vi "Compare FPGA.vi"(8 "error in (no error)":errorcluster, 10 "UDV Container":refnum<k21>[](array[refnum]), 11 "FPGA in":T1[](array[typedef]) {"UDVs"."To FPGA"."VS ref" format="%.0x"; "UDVs"."From FPGA"."VS ref" format="%.0x"; "VS ref" format="%.0x"; "Output Data"."BD Refs"."Data Reference" format="%.0x"; "Input Data"."BD Refs"."Data Reference" format="%.0x"}) -> (0 "error out":errorcluster, 3 "FPGA out":T1[](array[typedef]) {"UDVs"."To FPGA"."VS ref" format="%.0x"; "UDVs"."From FPGA"."VS ref" format="%.0x"; "VS ref" format="%.0x"; "Output Data"."BD Refs"."Data Reference" format="%.0x"; "Input Data"."BD Refs"."Data Reference" format="%.0x"})   [LabVIEW 2019, in "SEECD Engine.lvlib"]
uses:
  SEECD Engine.lvlib
  Type Defs/FPGA Data.ctl
  <vilib>/NI VeriStand/Custom Device API/Custom Device Item Ref.ctl
  Type Defs/Input Data.ctl
  <vilib>/NI VeriStand/Custom Device API/Block Data Reference.ctl
  <vilib>/NI VeriStand/Custom Device API/Data Reference.ctl
  Type Defs/Output Data.ctl
  Type Defs/UDV Data.ctl
  Type Defs/UDV Data Type.ctl
  Type Defs/FXP Config.ctl
  Shared/Globals/Error Strings.vi
  <resource>/objmgr/ni.var.rc
  <vilib>/NI VeriStand/Custom Device API/Custom Device API.lvlib
  Shared/SEECD Shared.lvlib
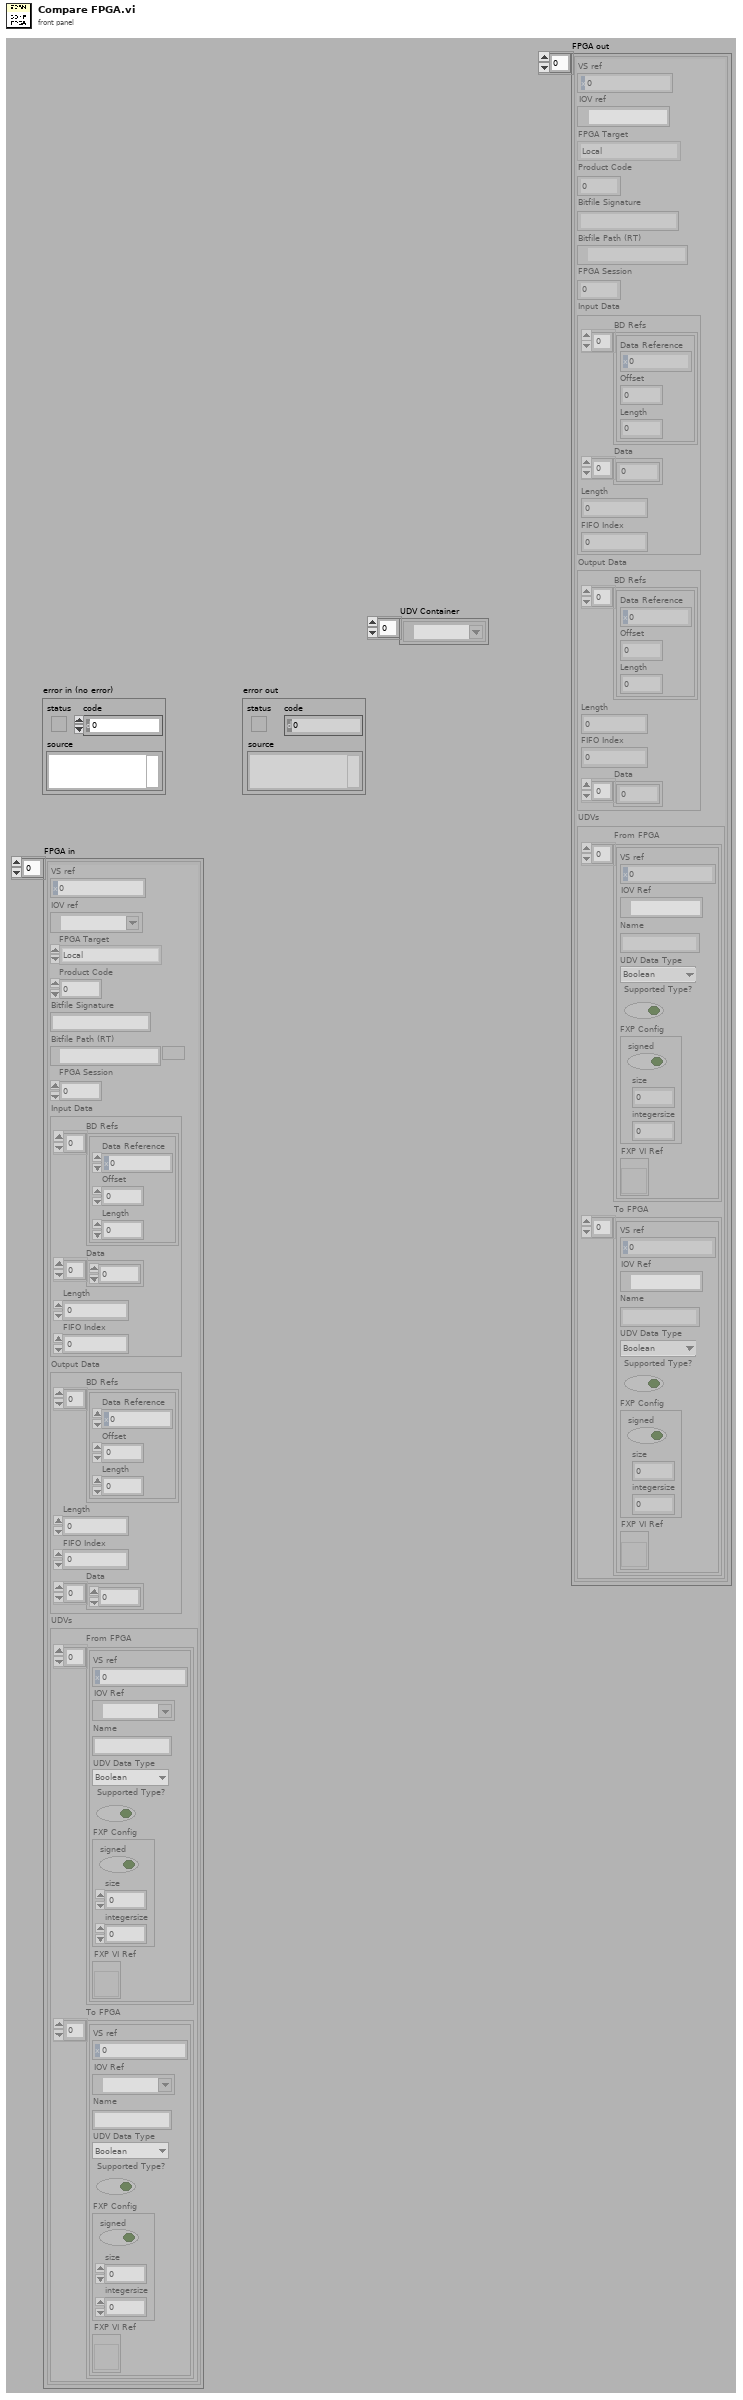
[diagram p1: front panel]
types:
  T1 = typedef "SEECD Engine.lvlib/FPGA Data.ctl" = cluster{"VS ref":T2, "IOV ref":refnum<k21>, "FPGA Target":enum16{"Local", "EtherCAT"}, "Product Code":u32, "Bitfile Signature":string, "Bitfile Path (RT)":path, "FPGA Session":u32, "Input Data":T3, "Output Data":T6, "UDVs":cluster{"From FPGA":T7[], "To FPGA":T7[]}}
  T2 = typedef "Custom Device API.lvlib/Custom Device Item Ref.ctl" = u64
  T3 = typedef "SEECD Engine.lvlib/Input Data.ctl" = cluster{"BD Refs":T4[], "Data":dbl[], "Length":i32, "FIFO Index":i32}
  T4 = typedef "Custom Device API.lvlib/Block Data Reference.ctl" = cluster{"Data Reference":T5, "Offset":u64, "Length":u64}
  T5 = typedef "Custom Device API.lvlib/Data Reference.ctl" = i32
  T6 = typedef "SEECD Engine.lvlib/Output Data.ctl" = cluster{"BD Refs":T4[], "Length":i32, "FIFO Index":i32, "Data":dbl[]}
  T7 = typedef "SEECD Engine.lvlib/UDV Data.ctl" = cluster{"VS ref":T2, "IOV Ref":refnum<k21>, "Name":string, "UDV Data Type":T8, "Supported Type?":bool, "FXP Config":T9, "FXP VI Ref":refnum<vi>}
  T8 = typedef "SEECD Engine.lvlib/UDV Data Type.ctl" = enum16{"Boolean", "Fixed Point", "Int8", "Int16", "Int32", "Int64", "U32 Bit Field", "UInt8", "UInt16", "UInt32", "UInt64", "Other", "DBL", "SGL"}
  T9 = typedef "SEECD Engine.lvlib/FXP Config.ctl" = cluster{"signed":bool, "size":u32, "integersize":i32}
  T10 = typedef "Custom Device API.lvlib/Custom Device Item Info.ctl" = cluster{"Name":string, "Is Channel":bool, "GUID":string, "Is Waveform":bool}
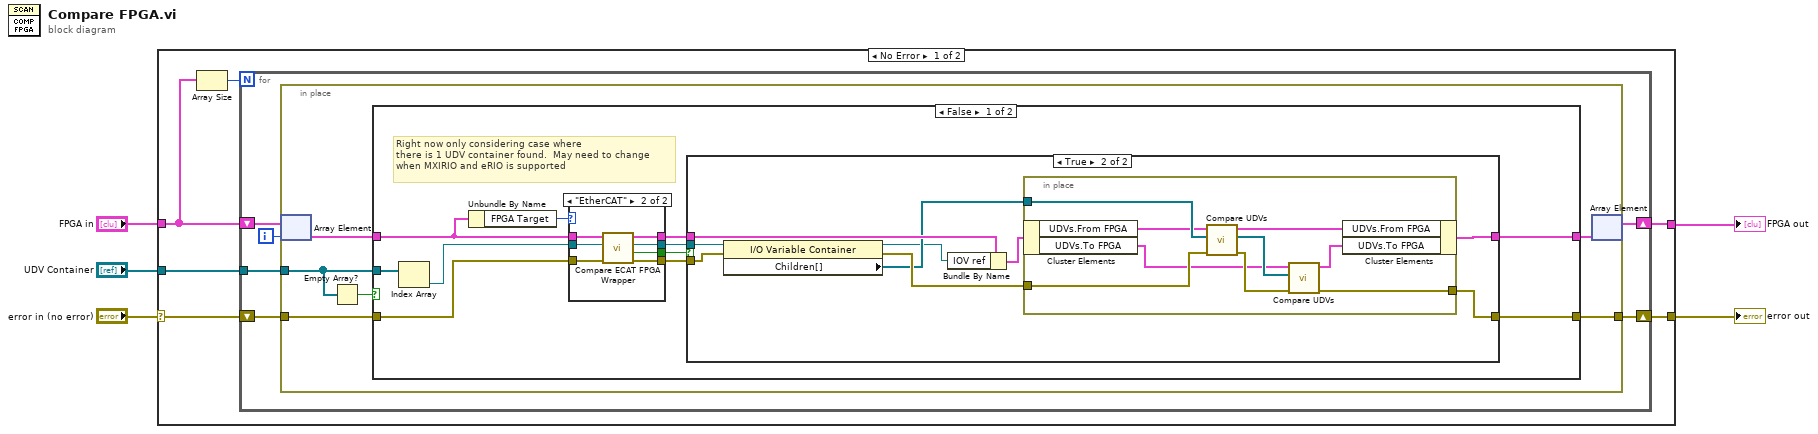
[diagram p0: block diagram]
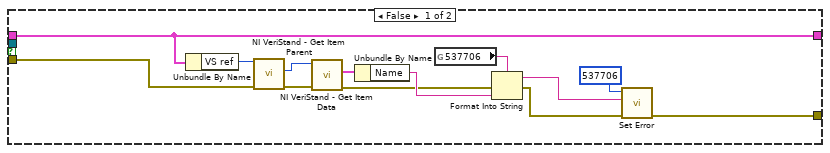
[diagram p2: hidden frame]
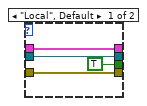
[diagram p3: hidden frame]
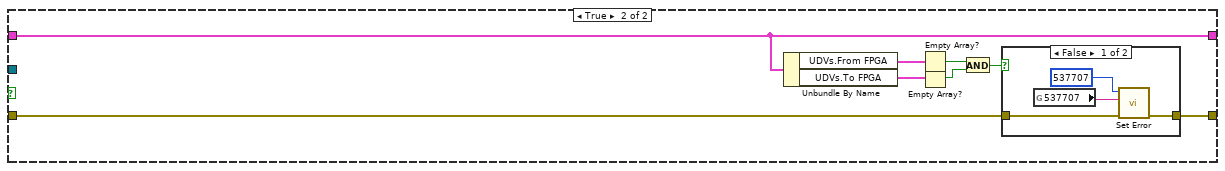
[diagram p4: hidden frame]
diagram:
  n1 = case shown="No Error" "error in (no error)" {
    selector: "error in (no error)" -> [w11 w91]
    tunnel: [w9 w91] -> w4
    tunnel: "FPGA in" -> [w7 w90]
    tunnel: "UDV Container" -> [w10 _]
    tunnel: [w6 w90] -> w1
    frame No Error {
      n2 = Array Size(array=w7) -> (size(s)=w8:i32)
      n3 = for {
        N: w8 -> [_]
        tunnel: w10 -> [w17]
        shift-right: [w13] -> w9
        shift-left: w11 -> [w16]
        shift-right: [w12] -> w6
        shift-left: w7 -> [w15]
        i -> [w14]
        n4 = in-place {
          in-place-border: w17 -> [w22]
          in-place-border: w16 -> [w21]
          in-place-border: [w18] -> w13
          n5 = in-place-array #1(w15, w14) -> (w20:T1)
          n6 = Empty Array?(array=w22) -> (empty?=w23:bool)
          n7 = case shown="False" w23 {
            tunnel: w20 -> [w32 w82]
            tunnel: w22 -> [w31 _]
            tunnel: w21 -> [w29 w83]
            tunnel: [w25 w82] -> w19
            tunnel: [w24 w84] -> w18
            frame False {
              # "Right now only considering case where\nthere is 1 UDV container found.  May need to change\nwhen MXIRIO and eRIO is supported"
              n8 = Index Array(array=w31) -> (element=w30:refnum<k21>)  [unwired: 1 in]
              n9 = Unbundle By Name(w32) -> ("FPGA Target"=w34:enum16{"Local", "EtherCAT"})
              n10 = case shown="\"EtherCAT\"" w34 {
                tunnel: w32 -> [w66 w75]
                tunnel: [TRUE w72] -> w33
                tunnel: w30 -> [w67 w76]
                tunnel: w29 -> [w68 w70]
                tunnel: [w68 w73] -> w28
                tunnel: [w67 w71] -> w27
                tunnel: [w66 w74] -> w26
                frame "Local", Default {
                }
                frame "EtherCAT" {
                  n11 = call "Compare ECAT FPGA Wrapper.vi"("error in (no error)"=w70, "UDV Container in"=w76, "FPGA in"=w75) -> ("error out"=w73:errorcluster, "Same?"=w72:bool, "UDV Container out"=w71:refnum<k21>, "FPGA out"=w74:T1)  [unwired: 5 in]
                }
              }
              n12 = case shown="True" w33 {
                tunnel: w26 -> [w47 w56]
                tunnel: w28 -> [w42 w54]
                tunnel: w27 -> [_ w55]
                tunnel: [w47 w50] -> w25
                tunnel: [w36 w49] -> w24
                frame False {
                  n13 = Unbundle By Name(w47) -> ("VS ref"=w46:T2)
                  n14 = call <vilib>:"NI VeriStand - Get Item Parent.vi"("error in (no error)"=w42, "Item Ref in"=w46) -> ("error out"=w44:errorcluster, "Parent Ref"=w45:T2)  [unwired: 6 in, 2 out]
                  n15 = call <vilib>:"NI VeriStand - Get Item Data.vi"("error in (no error)"=w44, "Item Ref in"=w45) -> ("error out"=w40:errorcluster, "Item Info"=w43:T10)  [unwired: 6 in, 2 out]
                  n16 = Unbundle By Name(w43) -> ("Name"=w41:string)
                  n17 = global read "Error Strings.vi" "537706"() -> (w39:string)
                  n18 = Format Into String(format string=w39, error in=w40, w41) -> (resulting string=w35:string, error out=w37:errorcluster)  [unwired: 1 in]
                  n19 = call "Set Error.vi"("error in (no error)"=w37, "Message"=w35, "Code"=537706) -> ("error out"=w36:errorcluster)  [unwired: 8 in]
                }
                frame True {
                  n20 = property class="I/O Variable Container"(reference=w55, error in=w54) -> (reference out=w48:refnum<k21>, error out=w53:errorcluster, "Children[]"=w52:refnum<k21>[])
                  n21 = Bundle By Name(cluster=w56, "IOV ref"=w48) -> (w51:T1)
                  n22 = in-place {
                    in-place-border: w53 -> [w65]
                    in-place-border: w52 -> [w64]
                    in-place-border: [w57] -> w49
                    n23 = in-place-cluster #2(w51) -> ("UDVs.From FPGA"=w61:T7[], "UDVs.To FPGA"=w60:T7[])
                    n24 = call "Compare UDVs.vi"("error in (no error)"=w65, "UDV refs in"=w64, "UDVs in"=w61) -> ("error out"=w62:errorcluster, "UDV refs out"=w63:refnum<k21>[], "UDVs out"=w59:T7[])  [unwired: 6 in]
                    n25 = call "Compare UDVs.vi"("error in (no error)"=w62, "UDV refs in"=w63, "UDVs in"=w60) -> ("error out"=w57:errorcluster, "UDVs out"=w58:T7[])  [unwired: 6 in, 1 out]
                    n26 = in-place-cluster #2("UDVs.From FPGA"=w59, "UDVs.To FPGA"=w58) -> (w50:T1)
                  }
                }
              }
            }
            frame True {
              n27 = Unbundle By Name(w82) -> ("UDVs.From FPGA"=w81:T7[], "UDVs.To FPGA"=w80:T7[])
              n28 = Empty Array?(array=w81) -> (empty?=w79:bool)
              n29 = Empty Array?(array=w80) -> (empty?=w78:bool)
              n30 = And(x=w79, y=w78) -> (x .and. y?=w77:bool)
              n31 = case shown="False" w77 {
                tunnel: [w88 w89] -> w84
                tunnel: w83 -> [w87 w89]
                frame False {
                  n32 = global read "Error Strings.vi" "537707"() -> (w86:string)
                  n33 = call "Set Error.vi"("error in (no error)"=w87, "Message"=w86, "Code"=537707 ("error code (0)")) -> ("error out"=w88:errorcluster)  [unwired: 8 in]
                }
                frame True {
                }
              }
            }
          }
          n34 = in-place-array #1(w19) -> (w12:T1[])  [unwired: 1 out]
        }
      }
    }
    frame Error {
    }
  }
  "error out" <- w4
  "FPGA out" <- w1
